vi "Lab2.vi"() -> ()   [LabVIEW 2011]
panel:
  out "Produsul numerelor - reprezentare tip Meter":dbl(knob) scale=0.0..10000.0
  out "Suma numerelor - reprezentare tip Tank":dbl(slide) scale=0.0..200.0 scale format="%#.2g"
  out "Produs":dbl
  out "Suma":dbl
  out "Numar2":dbl
  out "Numar1":dbl
  in  "Numarul 2":dbl(slide)=40.22346368715083 scale=0.0..100.0 scale format="%#.2g"
  in  "Numarul 1":dbl(slide)=20.670391061452513 scale=0.0..100.0 scale format="%#.2g"
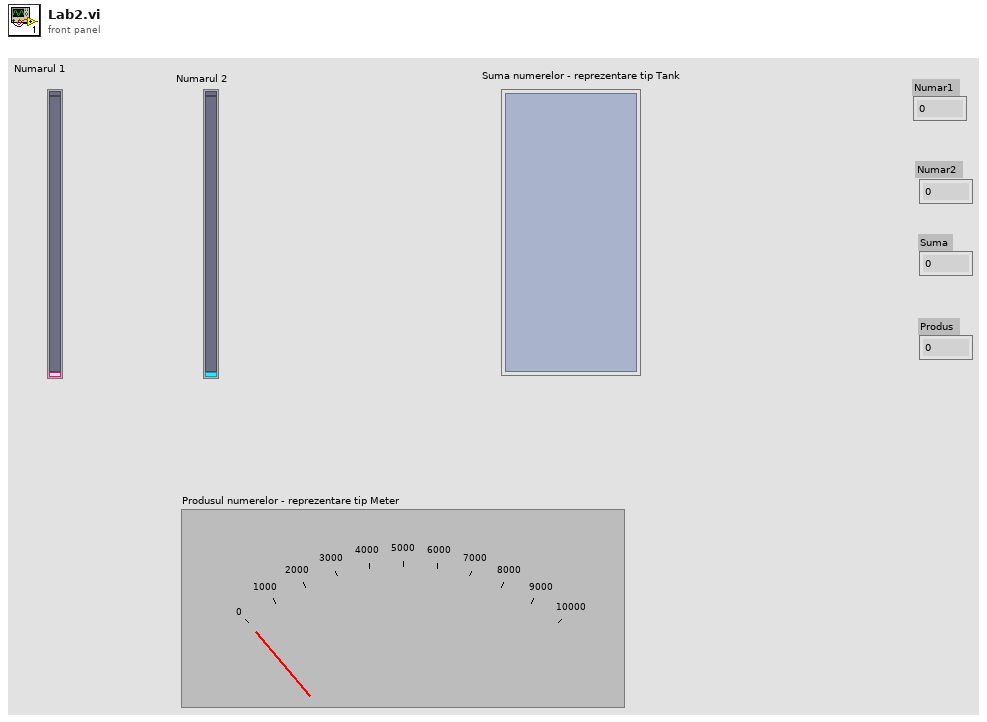
[diagram p1: front panel]
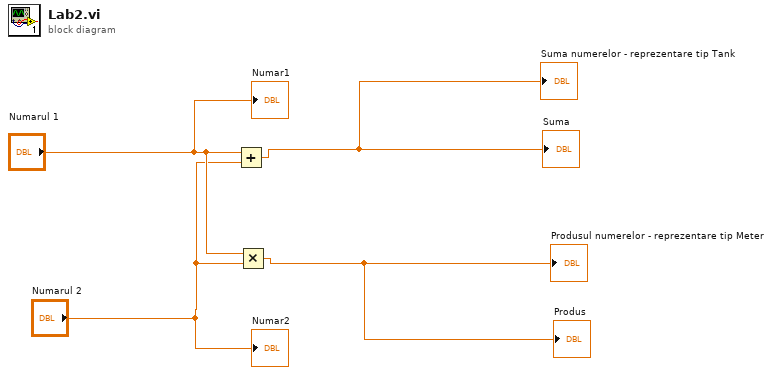
[diagram p0: block diagram]
diagram:
  n1 = Add(x="Numarul 1", y="Numarul 2") -> (x+y=→"Suma" →"Suma numerelor - reprezentare tip Tank":dbl)
  n2 = Multiply(x="Numarul 1", y="Numarul 2") -> (x*y=→"Produs" →"Produsul numerelor - reprezentare tip Meter":dbl)
  "Numar1" <- "Numarul 1"
  "Numar2" <- "Numarul 2"
